vi "1 in 2 out.vi"() -> ()   [LabVIEW 2016]
uses:
  Modulation_Signals.ctl
  Modulation_types.ctl
  <vilib>/DAQmx/write.llb/DAQmx Write (Analog 1D Wfm NChan NSamp).vi
  <vilib>/DAQmx/read.llb/DAQmx Read (Analog Wfm 1Chan NSamp).vi
  <vilib>/DAQmx/create/channels.llb/DAQmx Create Channel (AO-Voltage-Basic).vi
  <vilib>/DAQmx/create/channels.llb/DAQmx Create Channel (AI-Voltage-Basic).vi
  <vilib>/DAQmx/configure/timing.llb/DAQmx Timing (Sample Clock).vi
  <vilib>/DAQmx/miscellaneous.llb/DAQmx Fill In Error Info.vi
  <vilib>/Utility/config.llb/Write Key (String).vi
  <vilib>/Utility/config.llb/Write Key (Double).vi
  <vilib>/Utility/config.llb/Write Key (Path).vi
  <vilib>/Utility/config.llb/Write Key (Boolean).vi
  <vilib>/Utility/config.llb/Write Key (I32).vi
  <vilib>/Utility/file.llb/Write Delimited Spreadsheet (string).vi
  <vilib>/Utility/file.llb/Write Delimited Spreadsheet (DBL).vi
  <vilib>/Utility/config.llb/NI_LVConfig.lvlib
panel:
  in  "Signal param 2":dbl format="%#_6p"
  in  "Mearurement range":dbl=5.0 format="%0.2f"
  in  "High cutoff":dbl=20000.0 format="%#_13p"
  in  "Low cutoff":dbl=20.0 format="%#_13p"
  in  "Filter":bool=TRUE
  out "Export path":path
  in  "Export data":bool
  out "Sampling number":i32
  out "Iteration":i32
  out "Running":bool
  in  "Resampled iterations":dbl=1.0
  in  "Continious iterations":dbl=1.0
  in  "File path":path
  in  "Start":bool
  in  "Stop":bool
  in  "Modulation type":T1=enum."Simple"
  in  "Modulation signal":T2=enum."Sine"
  out "Output":waveform(dbl)[](graph)
  in  "Modulation depth":dbl=0.8 min=0.0 max=1.0 step=0.1 format="%0.2f"
  in  "Samples":dbl=200.0 format="%#_12g"
  in  "Signal frequency":dbl=1000.0 format="%#_6p"
  in  "Output Fs":dbl=192000.0 format="%#_6p"
  out "Samples per cycle":dbl=10.0
  in  "Carrier frequency":dbl=40000.0 min=0.0 step=1000.0 format="%#_6p"
  out "data":waveform(dbl)(graph) caption="Input"
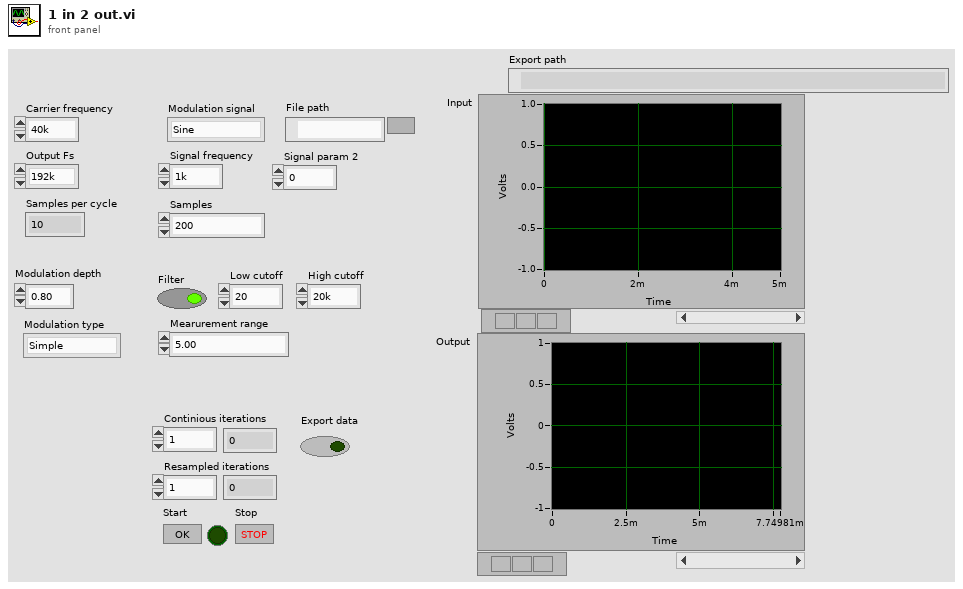
[diagram p1: front panel]
types:
  T1 = typedef "Modulation_types.ctl" = enum16{"None", "Add", "Simple", "Offset", "Square root", "Exponential"}
  T2 = typedef "Modulation_Signals.ctl" = enum16{"None", "Sine", "Chirp", "White Noise", "File"}
  T3 = typedef "NI_LVConfig.lvlib/Config Data RefNum.ctl" = refnum<k1>
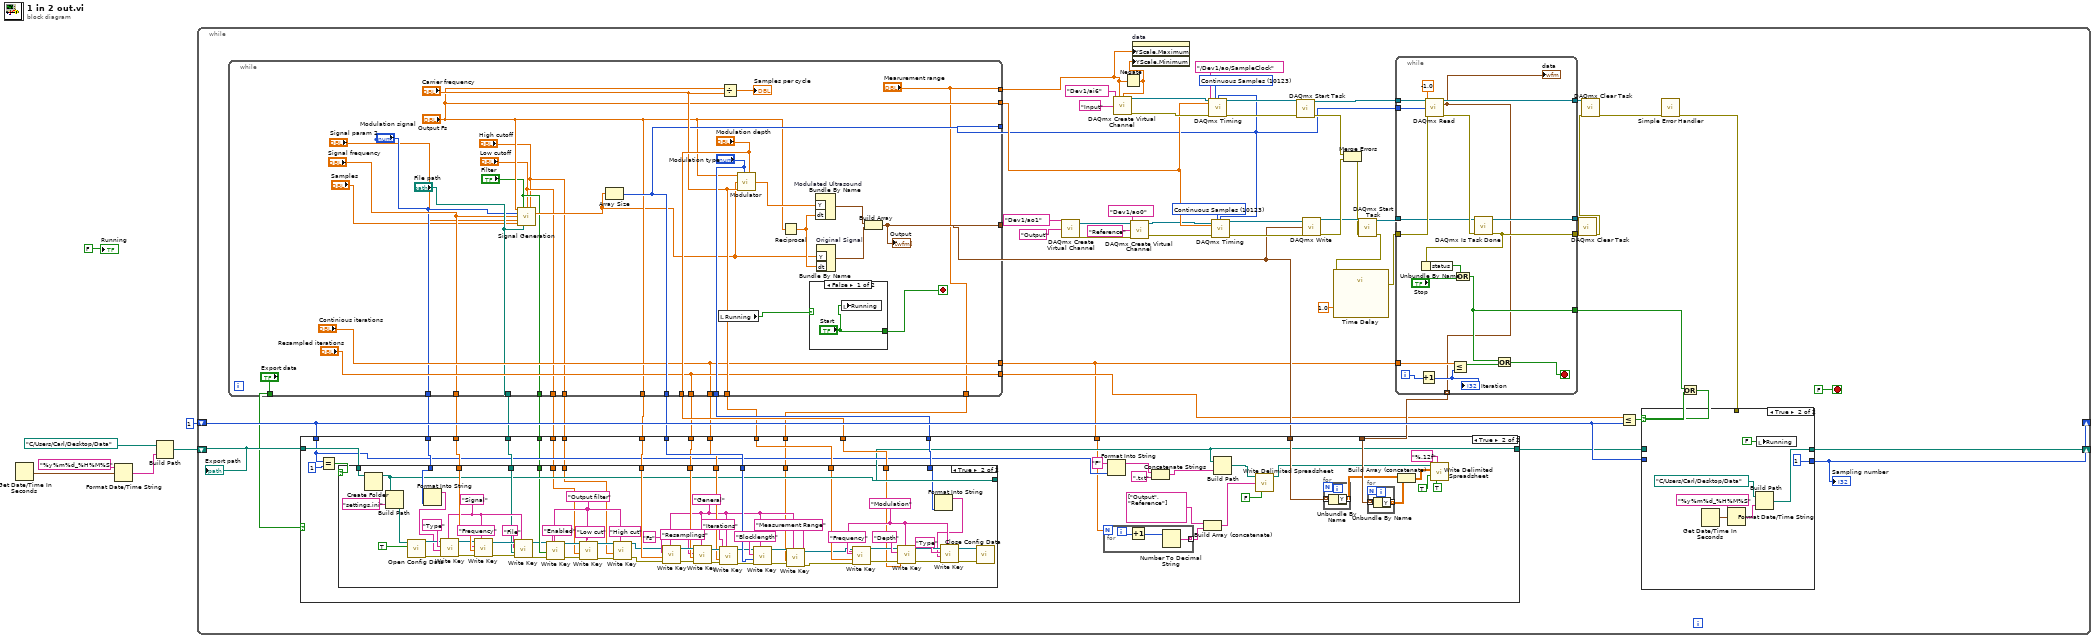
[diagram p0: block diagram]
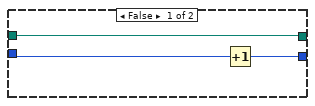
[diagram p4: hidden frame]
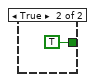
[diagram p5: hidden frame]
diagram:
  n1 = Get Date/Time In Seconds() -> (seconds since 1Jan1904=w6:timestamp)
  n2 = Format Date/Time String(time format string (%c)="%y%m%d_%H%M%S", seconds (now)=w6) -> (date/time string=w5:string)  [unwired: 1 in]
  n3 = Build Path(base path=path "C:/Users/Carl/Desktop/Data", name or relative path=w5) -> (appended path=w2:path)
  n4 = while {
    shift-right: [w40] -> _
    shift-left: 1 ("Sampling number") -> [w36]
    shift-right: [w34] -> _
    shift-left: w2 -> [w33]
    stop <- FALSE stop-if-true
    w64 = 10123 items=["Finite Samples"=10178, "Continuous Samples"=10123, "Hardware Timed Single Point"=12522] ("sample mode")
    w65 = 10123 items=["Finite Samples"=10178, "Continuous Samples"=10123, "Hardware Timed Single Point"=12522] ("sample mode")
    n5 = while {
      tunnel: [w232] -> w48
      tunnel: ["Output Fs"] -> w66
      tunnel: [w240] -> w21
      tunnel: ["Resampled iterations"] -> w12
      tunnel: ["Modulation depth"] -> w32
      tunnel: ["Modulation type"] -> w31
      tunnel: ["Modulation signal"] -> w30
      tunnel: ["Signal frequency"] -> w29
      tunnel: ["File path"] -> w28
      tunnel: ["Carrier frequency"] -> w27
      tunnel: ["Output Fs"] -> w26
      tunnel: [w232] -> w25
      tunnel: ["Resampled iterations"] -> w24
      tunnel: ["Continious iterations"] -> w11
      tunnel: ["Continious iterations"] -> w23
      tunnel: ["Export data"] -> w22
      tunnel: ["Mearurement range"] -> w18
      tunnel: ["Mearurement range"] -> w17
      tunnel: ["Filter"] -> w16
      tunnel: ["Low cutoff"] -> w15
      tunnel: ["High cutoff"] -> w14
      stop <- w237 stop-if-true
      n6 = call "Signal Generation.vi"("Output Fs"="Output Fs", "Filter"="Filter", "Low cutoff"="Low cutoff", "High cutoff"="High cutoff", "Signal Type"="Modulation signal", "Frequency 1"="Signal frequency", "Frequency 2"="Signal param 2", "Samples"="Samples", "File path"="File path") -> ("Output Signal"=w224:dbl[])  [unwired: 6 in]
      n7 = Array Size(array=w224) -> (size(s)=w232:i32)
      n8 = local read "Running"() -> (w236:bool)
      n9 = Divide(x="Output Fs", y="Carrier frequency") -> (x/y=→"Samples per cycle":dbl)
      n10 = call "Modulator.vi"("Sampling frequency"="Output Fs", "Modulation Type"="Modulation type", "Input Signal"=w224, "Carrier Frequency"="Carrier frequency", "Modulation depth"="Modulation depth") -> ("Output signal"=w241:dbl[])  [unwired: 4 in]
      n11 = Reciprocal(x="Output Fs") -> (1/x=w242:dbl)
      n12 = case shown="False" w236 {
        tunnel: ["Start" TRUE ("Start")] -> w237
        frame False {
          n13 = local write "Running"("Start") -> ()
        }
        frame True {
        }
      }
      n14 = Bundle By Name "Modulated Ultrasound"("Y"=w241, "dt"=w242) -> (w238:waveform(dbl))  [unwired: 1 in]
      n15 = Bundle By Name "Original Signal"("Y"=w224, "dt"=w242) -> (w243:waveform(dbl))  [unwired: 1 in]
      n16 = Build Array(w238, w243) -> (w240:waveform(dbl)[])
      "Output" <- w240
    }
    n17 = call-poly <vilib>:"DAQmx Create Virtual Channel.vi"("physical channels"=tag "Dev1/ao1", "name to assign"="Output") -> ("task out"=w47:refnum<k21>, "error out"=w44:errorcluster)  [unwired: 12 in]
    n18 = Negate(x=w18) -> (-x=w19:dbl)
    n19 = call-poly <vilib>:"DAQmx Create Virtual Channel.vi"("maximum value"=w18, "minimum value"=w19, "physical channels"=tag "Dev1/ai6", "name to assign"="Input") -> ("task out"=w69:refnum<k21>, "error out"=w68:errorcluster)  [unwired: 10 in]
    n20 = call-poly <vilib>:"DAQmx Create Virtual Channel.vi"("task in"=w47, "physical channels"=tag "Dev1/ao0", "name to assign"="Reference", "error in"=w44) -> ("task out"=w46:refnum<k21>, "error out"=w45:errorcluster)  [unwired: 10 in]
    n21 = property on="data" class="WFGraph (strict)"("YScale.Maximum"=w18, "YScale.Minimum"=w19) -> ()  [unwired: 2 in, 2 out]
    n22 = call-poly <vilib>:"DAQmx Timing.vi"("task/channels in"=w69, "sample mode"=w65, "samples per channel"=w48, "rate"=w66, "source"=tag "/Dev1/ao/SampleClock", "error in"=w68) -> ("task out"=w61:refnum<k21>, "error out"=w60:errorcluster)  [unwired: 8 in]
    n23 = call-poly <vilib>:"DAQmx Timing.vi"("task/channels in"=w46, "sample mode"=w64, "samples per channel"=w48, "rate"=w66, "error in"=w45) -> ("task out"=w62:refnum<k21>, "error out"=w63:errorcluster)  [unwired: 9 in]
    n24 = call <vilib>:"DAQmx Start Task.vi"("task/channels in"=w61, "error in"=w60) -> ("task out"=w55:refnum<k21>, "error out"=w59:errorcluster)  [unwired: 12 in]
    n25 = call-poly <vilib>:"DAQmx Write.vi"("task/channels in"=w62, "data"=w21, "error in"=w63) -> ("task out"=w57:refnum<k21>, "error out"=w58:errorcluster)  [unwired: 10 in, 1 out]
    n26 = Merge Errors(w59, w58) -> (w56:errorcluster)
    n27 = call <vilib>:"DAQmx Start Task.vi"("task/channels in"=w57, "error in"=w56) -> ("task out"=w54:refnum<k21>, "error out"=w10:errorcluster)  [unwired: 12 in]
    n28 = call "Time Delay"("error in (no error)"=w10, "Delay Time (s)"=1.0) -> ("error out"=w9:errorcluster)  [unwired: 9 in]
    n29 = while {
      tunnel: w48 -> [w212]
      tunnel: w55 -> [w217]
      tunnel: [w211] -> w53
      tunnel: w54 -> [w214]
      tunnel: [w213] -> w51
      tunnel: w9 -> [w216]
      tunnel: [w210] -> w50
      tunnel: [w201] -> w20 mode=indexing
      tunnel: [w203] -> w37
      tunnel: w11 -> [w202]
      i -> [w205]
      stop <- w207 stop-if-true
      n30 = Increment(x=w205) -> (x+1=w204:i32)
      "Iteration" <- w204
      n31 = call-poly <vilib>:"DAQmx Read.vi"("task/channels in"=w217, "number of samples per channel"=w212, "timeout"=-1.0, "error in"=w216) -> ("task out"=w211:refnum<k21>, "data"=w201:waveform(dbl), "error out"=w215:errorcluster)  [unwired: 9 in]
      "data" <- w201
      n32 = Less Or Equal?(x=w202, y=w204) -> (x <= y?=w206:bool)
      n33 = call <vilib>:"DAQmx Is Task Done.vi"("task/channels in"=w214, "error in"=w215) -> ("task out"=w213:refnum<k21>, "error out"=w210:errorcluster)  [unwired: 11 in, 1 out]
      n34 = Unbundle By Name(w210) -> ("status"=w209:bool)
      n35 = Or(x=w209, y="Stop") -> (x .or. y?=w203:bool)
      n36 = Or(x=w203, y=w206) -> (x .or. y?=w207:bool)
    }
    n37 = case shown="True" w22 {
      tunnel: w36 -> [_ w99]
      tunnel: w33 -> [w74 w100]
      tunnel: [w74 w89] -> w35
      tunnel: w32 -> [_ w110]
      tunnel: w31 -> [_ w109]
      tunnel: w30 -> [_ w108]
      tunnel: w29 -> [_ w107]
      tunnel: w28 -> [_ w106]
      tunnel: w27 -> [_ w105]
      tunnel: w26 -> [_ w104]
      tunnel: w25 -> [_ w103]
      tunnel: w24 -> [_ w102]
      tunnel: w23 -> [_ w101]
      tunnel: w21 -> [_ w95]
      tunnel: w20 -> [_ w93]
      tunnel: w17 -> [_ w87]
      tunnel: w16 -> [_ w86]
      tunnel: w15 -> [_ w85]
      tunnel: w14 -> [_ w84]
      tunnel: w11 -> [_ w83]
      frame False {
      }
      frame True {
        n38 = Equal?(x=w99, y=1) -> (x = y?=w111:bool)
        n39 = case shown="True" w111 {
          tunnel: w100 -> [w120 w146]
          tunnel: w110 -> [_ w131]
          tunnel: w109 -> [_ w150]
          tunnel: w108 -> [_ w152]
          tunnel: w107 -> [_ w177]
          tunnel: w106 -> [_ w170]
          tunnel: w105 -> [_ w130]
          tunnel: w104 -> [_ w167]
          tunnel: w103 -> [_ w166]
          tunnel: w102 -> [_ w162]
          tunnel: w101 -> [_ w158]
          tunnel: [w120 w145] -> w89
          tunnel: w87 -> [_ w140]
          tunnel: w86 -> [_ w127]
          tunnel: w85 -> [_ w126]
          tunnel: w84 -> [_ w125]
          frame False {
          }
          frame True {
            w135 = "Output filter" ("section")
            w142 = "General"
            w173 = "Signal" ("section")
            w168 = "Modulation" ("section")
            n40 = Create Folder(path (use dialog)=w146) -> (created path=w145:path)  [unwired: 2 in, 2 out]
            n41 = Build Path(base path=w145, name or relative path="settings.ini") -> (appended path=w148:path)
            n42 = call <vilib>:"Open Config Data.vi"("create file if necessary (T)"=TRUE, "configuration file path"=w148) -> ("error out"=w179:errorcluster, "refnum"=w178:T3)  [unwired: 7 in, 1 out]
            n43 = Format Into String(w152) -> (resulting string=w151:string)  [unwired: 3 in, 1 out]
            n44 = call-poly <vilib>:"Write Key.vi"("section"=w173, "error in (no error)"=w179, "value"=w151, "key"="Type", "refnum"=w178) -> ("error out"=w175:errorcluster, "refnum out"=w174:T3)  [unwired: 4 in, 1 out]
            n45 = call-poly <vilib>:"Write Key.vi"("section"=w173, "error in (no error)"=w175, "value"=w177, "key"="Frequency", "refnum"=w174) -> ("error out"=w171:errorcluster, "refnum out"=w172:T3)  [unwired: 4 in, 1 out]
            n46 = call-poly <vilib>:"Write Key.vi"("section"=w173, "error in (no error)"=w171, "value"=w170, "key"="File", "refnum"=w172) -> ("error out"=w122:errorcluster, "refnum out"=w121:T3)  [unwired: 4 in, 1 out]
            n47 = call-poly <vilib>:"Write Key.vi"("section"=w135, "error in (no error)"=w122, "value"=w127, "key"="Enabled", "refnum"=w121) -> ("error out"=w139:errorcluster, "refnum out"=w138:T3)  [unwired: 4 in, 1 out]
            n48 = call-poly <vilib>:"Write Key.vi"("section"=w135, "error in (no error)"=w139, "value"=w126, "key"="Low cut", "refnum"=w138) -> ("error out"=w136:errorcluster, "refnum out"=w137:T3)  [unwired: 4 in, 1 out]
            n49 = call-poly <vilib>:"Write Key.vi"("section"=w135, "error in (no error)"=w136, "value"=w125, "key"="High cut", "refnum"=w137) -> ("error out"=w124:errorcluster, "refnum out"=w123:T3)  [unwired: 4 in, 1 out]
            n50 = call-poly <vilib>:"Write Key.vi"("section"=w142, "error in (no error)"=w124, "value"=w167, "key"="Fs", "refnum"=w123) -> ("error out"=w164:errorcluster, "refnum out"=w163:T3)  [unwired: 4 in, 1 out]
            n51 = call-poly <vilib>:"Write Key.vi"("section"=w142, "error in (no error)"=w164, "value"=w162, "key"="Resamplings", "refnum"=w163) -> ("error out"=w159:errorcluster, "refnum out"=w160:T3)  [unwired: 4 in, 1 out]
            n52 = call-poly <vilib>:"Write Key.vi"("section"=w142, "error in (no error)"=w159, "value"=w158, "key"="Iterations", "refnum"=w160) -> ("error out"=w156:errorcluster, "refnum out"=w155:T3)  [unwired: 4 in, 1 out]
            n53 = call-poly <vilib>:"Write Key.vi"("section"=w142, "error in (no error)"=w156, "value"=w166, "key"="Blocklength", "refnum"=w155) -> ("error out"=w144:errorcluster, "refnum out"=w143:T3)  [unwired: 4 in, 1 out]
            n54 = call-poly <vilib>:"Write Key.vi"("section"=w142, "error in (no error)"=w144, "value"=w140, "key"="Measurement Range", "refnum"=w143) -> ("error out"=w128:errorcluster, "refnum out"=w129:T3)  [unwired: 4 in, 1 out]
            n55 = call-poly <vilib>:"Write Key.vi"("section"=w168, "error in (no error)"=w128, "value"=w130, "key"="Frequency", "refnum"=w129) -> ("error out"=w184:errorcluster, "refnum out"=w185:T3)  [unwired: 4 in, 1 out]
            n56 = call-poly <vilib>:"Write Key.vi"("section"=w168, "error in (no error)"=w184, "value"=w131, "key"="Depth", "refnum"=w185) -> ("error out"=w182:errorcluster, "refnum out"=w181:T3)  [unwired: 4 in, 1 out]
            n57 = Format Into String(w150) -> (resulting string=w149:string)  [unwired: 3 in, 1 out]
            n58 = call-poly <vilib>:"Write Key.vi"("section"=w168, "error in (no error)"=w182, "value"=w149, "key"="Type", "refnum"=w181) -> ("error out"=w153:errorcluster, "refnum out"=w154:T3)  [unwired: 4 in, 1 out]
            n59 = call <vilib>:"Close Config Data.vi"("error in (no error)"=w153, "refnum"=w154) -> ()  [unwired: 8 in, 2 out]
          }
        }
        n60 = for {
          N: w83 -> [_]
          tunnel: [w113] -> w76 mode=indexing
          i -> [w115]
          n61 = Increment(x=w115) -> (x+1=w114:i32)
          n62 = Number To Decimal String(number=w114) -> (decimal integer string=w113:string)  [unwired: 1 in]
        }
        n63 = Format Into String(initial string="F", w99) -> (resulting string=w98:string)  [unwired: 2 in, 1 out]
        n64 = Concatenate Strings(w98, ".txt" ("string")) -> (w96:string)
        n65 = Build Array (concatenate)(string[] ["Output", "Reference"], w76) -> (w79:string[])
        n66 = Build Path(base path=w89, name or relative path=w96) -> (appended path=w81:path)
        n67 = call-poly <vilib>:"Write Delimited Spreadsheet.vi"("file path (dialog if empty)"=w81, "1D data"=w79, "transpose? (no:F)"=FALSE) -> ("new file path (Not A Path if cancelled)"=w80:path)  [unwired: 11 in, 1 out]
        n68 = for {
          tunnel: w95 -> [w119] mode=indexing
          tunnel: [w118] -> w91 mode=indexing
          n69 = Unbundle By Name(w119) -> ("Y"=w118:dbl[])
        }
        n70 = for {
          tunnel: w93 -> [w117] mode=indexing
          tunnel: [w116] -> w92 mode=indexing
          n71 = Unbundle By Name(w117) -> ("Y"=w116:dbl[])
        }
        n72 = Build Array (concatenate)(w91, w92) -> (w90:dbl[][])
        n73 = call-poly <vilib>:"Write Delimited Spreadsheet.vi"("file path (dialog if empty)"=w80, "format (%.3f)"="%.12f", "2D data"=w90, "append to file? (new file:F)"=TRUE, "transpose? (no:F)"=TRUE) -> ()  [unwired: 9 in, 2 out]
      }
    }
    n74 = call <vilib>:"DAQmx Clear Task.vi"("task in"=w51, "error in"=w50) -> ("error out"=w52:errorcluster)  [unwired: 13 in]
    n75 = call <vilib>:"DAQmx Clear Task.vi"("task in"=w53, "error in"=w52) -> ("error out"=w49:errorcluster)  [unwired: 13 in]
    n76 = Less Or Equal?(x=w12, y=w36) -> (x <= y?=w39:bool)
    n77 = call <vilib>:"Simple Error Handler.vi"("error in (no error)"=w49) -> ("error out"=w13:errorcluster)  [unwired: 4 in, 4 out]
    n78 = Or(x=w37, y=w39) -> (x .or. y?=w38:bool)
    n79 = case shown="True" w38 {
      tunnel: w36 -> [w192 _]
      tunnel: [w191 1 ("Sampling number")] -> w40
      tunnel: w13 -> [_ _]
      tunnel: [w190 w193] -> w34
      tunnel: w35 -> [w190 _]
      frame False {
        n80 = Increment(x=w192) -> (x+1=w191:i32)
      }
      frame True {
        n81 = Get Date/Time In Seconds() -> (seconds since 1Jan1904=w197:timestamp)
        n82 = Format Date/Time String(time format string (%c)="%y%m%d_%H%M%S", seconds (now)=w197) -> (date/time string=w196:string)  [unwired: 1 in]
        n83 = Build Path(base path=path "C:/Users/Carl/Desktop/Data", name or relative path=w196) -> (appended path=w193:path)
        n84 = local write "Running"(FALSE ("Running")) -> ()
      }
    }
    "Sampling number" <- w40
    "Export path" <- w33
  }
  "Running" <- FALSE
